vi "Analyze Pulse Waveform.vi"(0 "Waveform In":waveform(dbl)={"t0"=timestamp(3418839276.250478 s since 1904-01-01), "dt"=1e-06, "Y"=[5.0, 5.0, 9.0, 9.0, 9.0, 9.0, 9.0, 9.0, 9.0, 9.0, 5.0, 5.0, 5.0, 3.0, 3.0, 3.0, 3.0, 3.0, 3.0, 3.0, 3.0, 3.0, 3.0, 3.0, 3.0, 3.0, 3.0, 3.0, 3.0, 5.0, 5.0, 5.0, 5.0, 8.0, 8.0, 8.0, 8.0, 8.0, 8.0, 8.0, 8.0, 5.0, 5.0, 5.0, 3.0, 3.0, 3.0, 3.0, 3.0, 3.0, 3.0, 3.0, 3.0, 3.0, 3.0, 3.0, 3.0, 3.0, 3.0, 3.0, 5.0, 5.0, 5.0, 5.0, 0.0, 0.0, 0.0, 0.0, 0.0, 5.0, 5.0, 5.0, 5.0, 5.0, 5.0, 5.0, 5.0, 5.0, 5.0, 5.0, 5.0, 5.0, 5.0, 5.0, 5.0, 5.0, 5.0, 5.0, 5.0, 5.0, 5.0, 5.0, 5.0, 5.0, 5.0, 5.0, 5.0, 5.0, 5.0, 5.0, 5.0, 5.0, 9.0, 9.0, 9.0, 9.0, 9.0, 9.0, 9.0, 9.0, 5.0, 5.0, 5.0, 3.0, 3.0, 3.0, 3.0, 3.0, 3.0, 3.0, 3.0, 3.0, 3.0, 3.0, 3.0, 3.0, 3.0, 3.0, 3.0, 5.0, 5.0, 5.0, 5.0, 8.0, 8.0, 8.0, 8.0, 8.0, 8.0, 8.0, 8.0, 5.0, 5.0, 5.0, 3.0, 3.0, 3.0, 3.0, 3.0, 3.0, 3.0, 3.0, 3.0, 3.0, 3.0, 3.0, 3.0, 3.0, 3.0, 3.0, 5.0, 5.0, 5.0, 5.0, 0.0, 0.0, 0.0, 0.0, 0.0, 5.0, 5.0, 5.0, 5.0, 5.0, 5.0, 5.0, 5.0, 5.0, 5.0, 5.0, 5.0, 5.0, 5.0, 5.0, 5.0, 5.0, 5.0, 5.0, 5.0, 5.0, 5.0, 5.0, 5.0, 5.0, 5.0, 5.0, 5.0, 5.0, 5.0, 5.0, 5.0, 5.0, 9.0, 9.0, 9.0, 9.0, 9.0, 9.0, 9.0, 9.0, 5.0, 5.0, 5.0, 3.0, 3.0, 3.0, 3.0, 3.0, 3.0, 3.0, 3.0, 3.0, 3.0, 3.0, 3.0, 3.0, 3.0, 3.0, 3.0, 5.0, 5.0, 5.0, 5.0, 8.0, 8.0, 8.0, 8.0, 8.0, 8.0, 8.0, 8.0, 5.0, 5.0, 5.0, 3.0, 3.0, 3.0, 3.0, 3.0, 3.0, 3.0, 3.0, 3.0, 3.0, 3.0, 3.0, 3.0, 3.0, 3.0, 3.0, 5.0, 5.0, 5.0, 5.0, 0.0, 0.0, 0.0, 0.0, 0.0, 5.0, 5.0, 5.0, 5.0, 5.0, 5.0, 5.0, 5.0, 5.0, 5.0, 5.0, 5.0, 5.0, 5.0, 5.0, 5.0, 5.0, 5.0, 5.0, 5.0, 5.0, 5.0, 5.0, 5.0, 5.0, 5.0, 5.0, 5.0, 5.0, 5.0, 5.0, 5.0, 5.0, 9.0, 9.0, 9.0, 9.0, 9.0, 9.0, 9.0, 9.0, 5.0, 5.0, 5.0, 3.0, 3.0, 3.0, 3.0, 3.0, 3.0, 3.0, 3.0, 3.0, 3.0, 3.0, 3.0, 3.0, 3.0, 3.0, 3.0, 5.0, 5.0, 5.0, 5.0, 8.0, 8.0, 8.0, 8.0, 8.0, 8.0, 8.0, 8.0, 5.0, 5.0, 5.0, 3.0, 3.0, 3.0, 3.0, 3.0, 3.0, 3.0, 3.0, 3.0, 3.0, 3.0, 3.0, 3.0, 3.0, 3.0, 3.0, 5.0, 5.0, 5.0, 5.0, 0.0, 0.0, 0.0, 0.0, 0.0, 5.0, 5.0, 5.0, 5.0, 5.0, 5.0, 5.0, 5.0, 5.0, 5.0, 5.0, 5.0, 5.0, 5.0, 5.0, 5.0, 5.0, 5.0, 5.0, 5.0, 5.0, 5.0, 5.0, 5.0, 5.0, 5.0, 5.0, 5.0, 5.0, 5.0, 5.0, 5.0, 5.0, 9.0, 9.0, 9.0, 9.0, 9.0, 9.0, 9.0, 9.0, 5.0, 5.0, 5.0, 3.0, 3.0, 3.0, 3.0, 3.0, 3.0, 3.0, 3.0, 3.0, 3.0, 3.0, 3.0, 3.0, 3.0, 3.0, 3.0, 5.0, 5.0, 5.0, 5.0, 8.0, 8.0, 8.0, 8.0, 8.0, 8.0, 8.0, 8.0, 5.0, 5.0, 5.0, 3.0, 3.0, 3.0, 3.0, 3.0, 3.0, 3.0, 3.0, 3.0, 3.0, 3.0, 3.0, 3.0, 3.0, 3.0, 3.0, 5.0, 5.0, 5.0, 5.0, 0.0, 0.0, 0.0, 0.0, 0.0, 5.0, 5.0, 5.0, 5.0, 5.0, 5.0, 5.0, 5.0, 5.0, 5.0, 5.0, 5.0, 5.0, 5.0, 5.0, 5.0, 5.0, 5.0, 5.0, 5.0, 5.0, 5.0, 5.0, 5.0, 5.0, 5.0, 5.0, 5.0, 5.0, 5.0, 5.0, 5.0, 5.0, 5.0]}, 5 "Repetitions in the Input Waveform":i32, 7 "Pulse Characteristics":T1={"Pulses per Cycle"=2, "Load Resistance (Ohms)"=750.0, "Krec Value"=2, "Recovery Mode (T=Active)"=TRUE, "Target Stim Currents (Amps)"=[]}) -> (4 "Recovery Voltage":dbl[](array[numeric]), 6 "Recovery Holdoff Current":dbl[](array[numeric]), 8 "Interphase Delay Current":dbl[](array[numeric]), 10 "CBC Phase Voltage":dbl[](array[numeric]))   [LabVIEW 2010]
uses:
  <vilib>/measure/mamon.llb/Trigger Detection for 1 Channel.vi
  <vilib>/measure/NI_MAPro.lvlib
  <vilib>/Analysis/NI_AALBase.lvlib
panel:
  out "Normalized Waveform":waveform(dbl)(graph)
  # "The input waveform should be a capture of the STIM chip output\n(before the cap) when the output is held at 1/2 HVDD by the\nLoad Resistance.  This ensures that passive recovery and CBC\npulses are captured, because they look like pulses pulled to GND."
  # "The elements in these arrays correspond to the pulses per cycle.\nThey are the averages over all the repetitions in the waveform."
  # "Enter Target Current\nfor each in array below"
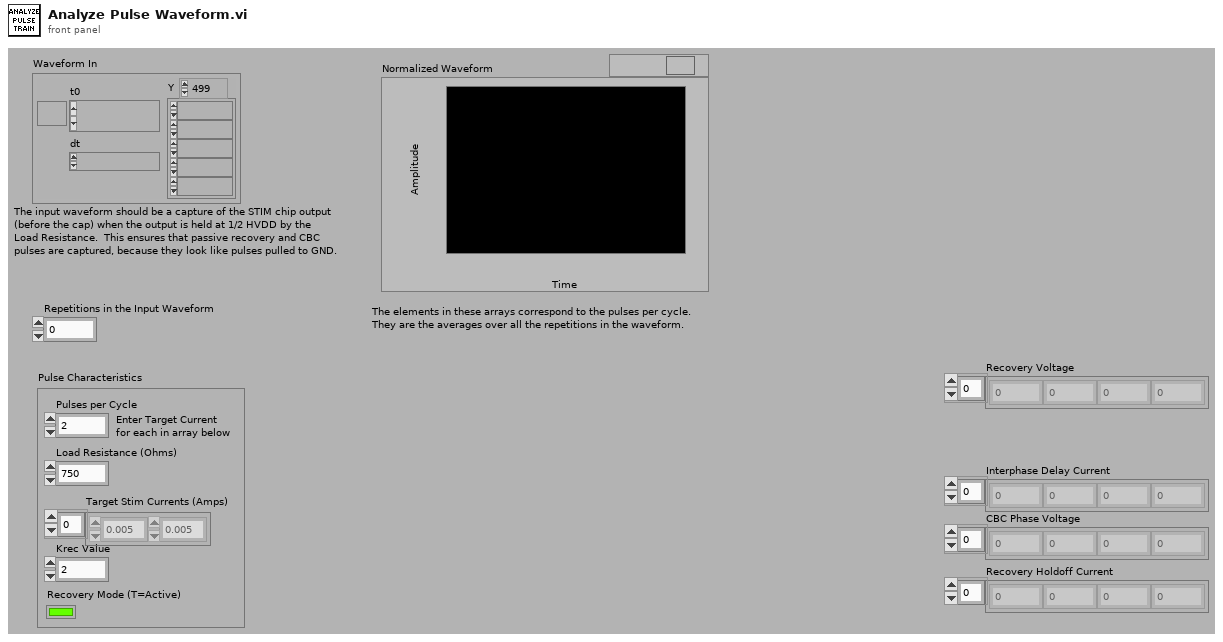
[diagram p1: front panel]
types:
  T1 = cluster{"Pulses per Cycle":i32, "Load Resistance (Ohms)":dbl, "Krec Value":i32, "Recovery Mode (T=Active)":bool, "Target Stim Currents (Amps)":dbl[]}
  T2 = cluster{"trigger slope":u16, "Trigger Level":dbl}[]
  T3 = cluster{"trigger slope":u16, "Trigger Level":dbl}
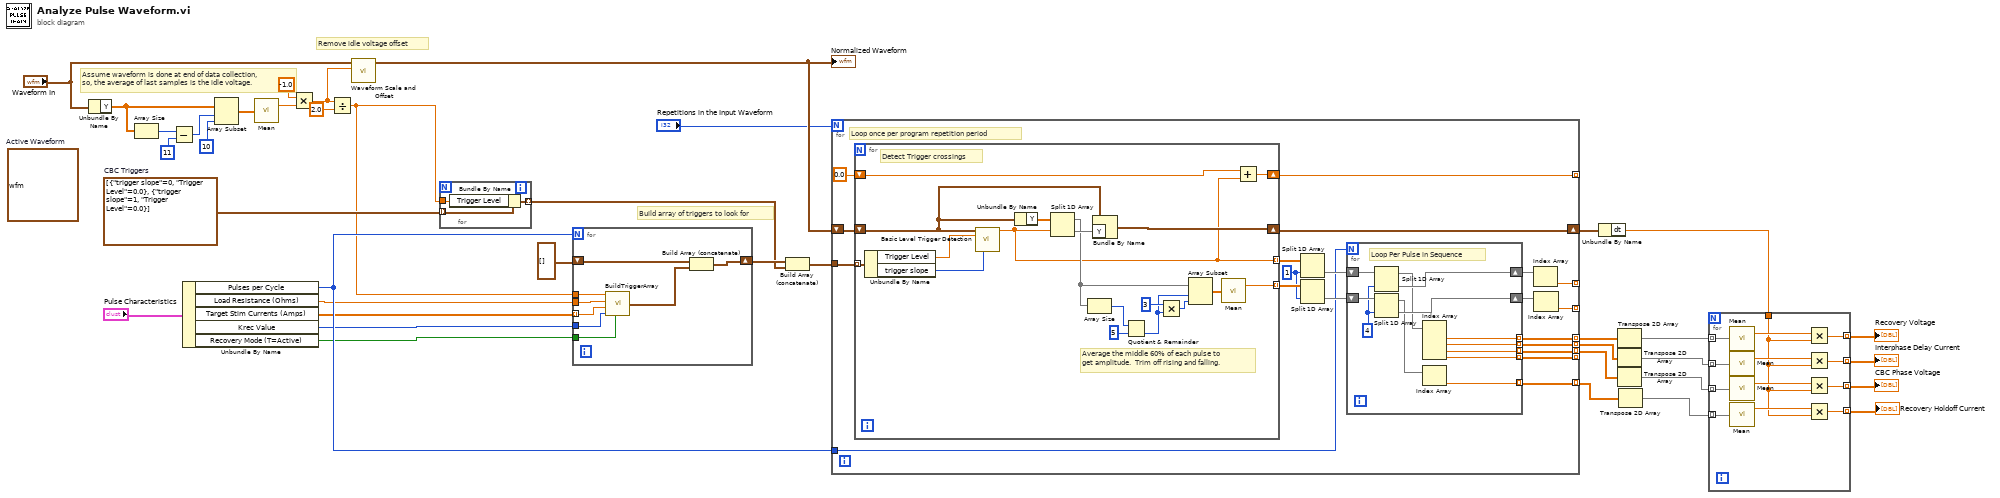
[diagram p0: block diagram]
diagram:
  (unwired) waveform(dbl) {"t0"=timestamp(3418839276.250478 s since 1904-01-01), "dt"=1e-06, "Y"=[5.0, 5.0, 9.0, 9.0, 9.0, 9.0, 9.0, 9.0, 9.0, 9.0, 5.0, 5.0, 5.0, 3.0, 3.0, 3.0, 3.0, 3.0, 3.0, 3.0, 3.0, 3.0, 3.0, 3.0, 3.0, 3.0, 3.0, 3.0, 3.0, 5.0, 5.0, 5.0, 5.0, 8.0, 8.0, 8.0, 8.0, 8.0, 8.0, 8.0, 8.0, 5.0, 5.0, 5.0, 3.0, 3.0, 3.0, 3.0, 3.0, 3.0, 3.0, 3.0, 3.0, 3.0, 3.0, 3.0, 3.0, 3.0, 3.0, 3.0, 5.0, 5.0, 5.0, 5.0, 0.0, 0.0, 0.0, 0.0, 0.0, 5.0, 5.0, 5.0, 5.0, 5.0, 5.0, 5.0, 5.0, 5.0, 5.0, 5.0, 5.0, 5.0, 5.0, 5.0, 5.0, 5.0, 5.0, 5.0, 5.0, 5.0, 5.0, 5.0, 5.0, 5.0, 5.0, 5.0, 5.0, 5.0, 5.0, 5.0, 5.0, 5.0, 9.0, 9.0, 9.0, 9.0, 9.0, 9.0, 9.0, 9.0, 5.0, 5.0, 5.0, 3.0, 3.0, 3.0, 3.0, 3.0, 3.0, 3.0, 3.0, 3.0, 3.0, 3.0, 3.0, 3.0, 3.0, 3.0, 3.0, 5.0, 5.0, 5.0, 5.0, 8.0, 8.0, 8.0, 8.0, 8.0, 8.0, 8.0, 8.0, 5.0, 5.0, 5.0, 3.0, 3.0, 3.0, 3.0, 3.0, 3.0, 3.0, 3.0, 3.0, 3.0, 3.0, 3.0, 3.0, 3.0, 3.0, 3.0, 5.0, 5.0, 5.0, 5.0, 0.0, 0.0, 0.0, 0.0, 0.0, 5.0, 5.0, 5.0, 5.0, 5.0, 5.0, 5.0, 5.0, 5.0, 5.0, 5.0, 5.0, 5.0, 5.0, 5.0, 5.0, 5.0, 5.0, 5.0, 5.0, 5.0, 5.0, 5.0, 5.0, 5.0, 5.0, 5.0, 5.0, 5.0, 5.0, 5.0, 5.0, 5.0, 9.0, 9.0, 9.0, 9.0, 9.0, 9.0, 9.0, 9.0, 5.0, 5.0, 5.0, 3.0, 3.0, 3.0, 3.0, 3.0, 3.0, 3.0, 3.0, 3.0, 3.0, 3.0, 3.0, 3.0, 3.0, 3.0, 3.0, 5.0, 5.0, 5.0, 5.0, 8.0, 8.0, 8.0, 8.0, 8.0, 8.0, 8.0, 8.0, 5.0, 5.0, 5.0, 3.0, 3.0, 3.0, 3.0, 3.0, 3.0, 3.0, 3.0, 3.0, 3.0, 3.0, 3.0, 3.0, 3.0, 3.0, 3.0, 5.0, 5.0, 5.0, 5.0, 0.0, 0.0, 0.0, 0.0, 0.0, 5.0, 5.0, 5.0, 5.0, 5.0, 5.0, 5.0, 5.0, 5.0, 5.0, 5.0, 5.0, 5.0, 5.0, 5.0, 5.0, 5.0, 5.0, 5.0, 5.0, 5.0, 5.0, 5.0, 5.0, 5.0, 5.0, 5.0, 5.0, 5.0, 5.0, 5.0, 5.0, 5.0, 9.0, 9.0, 9.0, 9.0, 9.0, 9.0, 9.0, 9.0, 5.0, 5.0, 5.0, 3.0, 3.0, 3.0, 3.0, 3.0, 3.0, 3.0, 3.0, 3.0, 3.0, 3.0, 3.0, 3.0, 3.0, 3.0, 3.0, 5.0, 5.0, 5.0, 5.0, 8.0, 8.0, 8.0, 8.0, 8.0, 8.0, 8.0, 8.0, 5.0, 5.0, 5.0, 3.0, 3.0, 3.0, 3.0, 3.0, 3.0, 3.0, 3.0, 3.0, 3.0, 3.0, 3.0, 3.0, 3.0, 3.0, 3.0, 5.0, 5.0, 5.0, 5.0, 0.0, 0.0, 0.0, 0.0, 0.0, 5.0, 5.0, 5.0, 5.0, 5.0, 5.0, 5.0, 5.0, 5.0, 5.0, 5.0, 5.0, 5.0, 5.0, 5.0, 5.0, 5.0, 5.0, 5.0, 5.0, 5.0, 5.0, 5.0, 5.0, 5.0, 5.0, 5.0, 5.0, 5.0, 5.0, 5.0, 5.0, 5.0, 9.0, 9.0, 9.0, 9.0, 9.0, 9.0, 9.0, 9.0, 5.0, 5.0, 5.0, 3.0, 3.0, 3.0, 3.0, 3.0, 3.0, 3.0, 3.0, 3.0, 3.0, 3.0, 3.0, 3.0, 3.0, 3.0, 3.0, 5.0, 5.0, 5.0, 5.0, 8.0, 8.0, 8.0, 8.0, 8.0, 8.0, 8.0, 8.0, 5.0, 5.0, 5.0, 3.0, 3.0, 3.0, 3.0, 3.0, 3.0, 3.0, 3.0, 3.0, 3.0, 3.0, 3.0, 3.0, 3.0, 3.0, 3.0, 5.0, 5.0, 5.0, 5.0, 0.0, 0.0, 0.0, 0.0, 0.0, 5.0, 5.0, 5.0, 5.0, 5.0, 5.0, 5.0, 5.0, 5.0, 5.0, 5.0, 5.0, 5.0, 5.0, 5.0, 5.0, 5.0, 5.0, 5.0, 5.0, 5.0, 5.0, 5.0, 5.0, 5.0, 5.0, 5.0, 5.0, 5.0, 5.0, 5.0, 5.0, 5.0, 5.0]}  # Active Waveform
  w27 = T2 [{"trigger slope"=0, "Trigger Level"=0.0}, {"trigger slope"=1, "Trigger Level"=0.0}]  # CBC Triggers
  # "Build array of triggers to look for"
  # "Remove idle voltage offset"
  # "Assume waveform is done at end of data collection,\nso, the average of last samples is the idle voltage."
  n1 = Unbundle By Name("Waveform In") -> ("Y"=w35:dbl[])
  n2 = Array Size(array=w35) -> (size(s)=w39:i32)
  n3 = Subtract(x=w39, y=11) -> (x-y=w37:i32)
  n4 = Unbundle By Name("Pulse Characteristics") -> ("Pulses per Cycle"=w15:i32, "Load Resistance (Ohms)"=w8:dbl, "Target Stim Currents (Amps)"=w12:dbl[], "Krec Value"=w11:i32, "Recovery Mode (T=Active)"=w13:bool)
  n5 = Array Subset(array=w35, index=w37, length=10 ("index")) -> (w34:dbl[])
  n6 = call <vilib>:"Mean.vi"("X"=w34) -> ("mean"=w33:dbl)  [unwired: 1 out]
  n7 = Multiply(x=-1.0, y=w33) -> (x*y=w26:dbl)
  n8 = Divide(x=w26, y=2.0) -> (x/y=w14:dbl)
  n9 = call <vilib>:"Waveform Scale and Offset.vi"("offset"=w26, "waveform in"="Waveform In") -> ("waveform out"=w22:waveform(dbl))  [unwired: 8 in, 1 out]
  "Normalized Waveform" <- w22
  n10 = for {
    tunnel: w27 -> [w42] mode=indexing
    tunnel: w14 -> [w41]
    tunnel: [w40] -> w24 mode=indexing
    n11 = Bundle By Name(cluster=w42, "Trigger Level"=w41) -> (w40:T3)
  }
  n12 = for {
    N: w15 -> [_]
    shift-right: [w50] -> w28
    shift-left: T2 [] -> [w49]
    tunnel: w14 -> [w48]
    tunnel: w13 -> [w47]
    tunnel: w8 -> [w46]
    tunnel: w12 -> [w45] mode=indexing
    tunnel: w11 -> [w44]
    n13 = call "BuildTriggerArray.vi"("CBC Trigger Level"=w48, "Load Resistance (Ohms)"=w46, "Target Stim Current (Amps)"=w45, "Krec Value"=w44, "Recovery Mode (T=Active)"=w47) -> ("Pulse Triggers"=w43:T2)
    n14 = Build Array (concatenate)(w49, w43) -> (w50:T2)
  }
  n15 = Build Array (concatenate)(w28, w24) -> (w23:T2)
  n16 = for {
    N: "Repetitions in the Input Waveform" -> [_]
    tunnel: w23 -> [w70]
    shift-right: [w66] -> w9
    shift-left: w22 -> [w69]
    tunnel: w15 -> [w63]
    tunnel: [w60] -> _ mode=indexing
    tunnel: [w59] -> _ mode=indexing
    tunnel: [w58] -> w21 mode=indexing
    tunnel: [w57] -> w20 mode=indexing
    tunnel: [w56] -> w19 mode=indexing
    tunnel: [w55] -> _ mode=indexing
    tunnel: [w52] -> _ mode=indexing
    tunnel: [w51] -> w1 mode=indexing
    w67 = 1 ("index")
    # "Loop once per program repetition period"
    n17 = for {
      tunnel: w70 -> [w100] mode=indexing
      shift-right: [w86] -> w66
      shift-left: w69 -> [w95]
      tunnel: [w87] -> w68 mode=indexing
      tunnel: [w83] -> w53 mode=indexing
      shift-right: [w85] -> w52
      shift-left: 0.0 -> [w84]
      # "Detect Trigger crossings"
      # "Average the middle 60% of each pulse to\nget amplitude.  Trim off rising and falling."
      n18 = Unbundle By Name(w100) -> ("Trigger Level"=w99:dbl, "trigger slope"=w98:u16)
      n19 = call-poly <vilib>:"Basic Level Trigger Detection.vi"("signal in"=w95, "level"=w99, "trigger slope"=w98) -> ("trigger location"=w83:dbl)  [unwired: 10 in, 2 out]
      n20 = Unbundle By Name(w95) -> ("Y"=w97:dbl[])
      n21 = Split 1D Array(array=w97, index=w83) -> (first subarray=w89:dbl[], second subarray=w96:dbl[])
      n22 = Array Size(array=w89) -> (size(s)=w94:i32)
      n23 = Bundle By Name(cluster=w95, "Y"=w96) -> (w86:waveform(dbl))
      n24 = Quotient & Remainder(x=w94, y=5) -> (floor(x/y)=w91:i32)  [unwired: 1 out]
      n25 = Multiply(x=3, y=w91) -> (x*y=w90:i32)
      n26 = Array Subset(array=w89, index=w91, length=w90) -> (w88:dbl[])
      n27 = call <vilib>:"Mean.vi"("X"=w88) -> ("mean"=w87:dbl)  [unwired: 1 out]
      n28 = Add(x=w84, y=w83) -> (x+y=w85:dbl)
    }
    n29 = Split 1D Array(array=w53, index=w67) -> (second subarray=w65:dbl[])  [unwired: 1 out]
    n30 = Split 1D Array(array=w68, index=w67) -> (second subarray=w64:dbl[])  [unwired: 1 out]
    n31 = for {
      N: w63 -> [_]
      shift-right: [w80] -> w62
      shift-left: w65 -> [w82]
      shift-right: [w79] -> w61
      shift-left: w64 -> [w81]
      tunnel: [w77] -> w58 mode=indexing
      tunnel: [w76] -> w57 mode=indexing
      tunnel: [w75] -> w56 mode=indexing
      tunnel: [w74] -> w55 mode=indexing
      tunnel: [w71] -> w51 mode=indexing
      w73 = 4 ("index")
      # "Loop Per Pulse in Sequence"
      n32 = Split 1D Array(array=w82, index=w73) -> (first subarray=w78:dbl[], second subarray=w80:dbl[])
      n33 = Split 1D Array(array=w81, index=w73) -> (first subarray=w72:dbl[], second subarray=w79:dbl[])
      n34 = Index Array(array=w78) -> (element #1=w77:dbl, element #2=w76:dbl, element #3=w75:dbl, element #4=w74:dbl)  [unwired: 4 in]
      n35 = Index Array(array=w72) -> (element=w71:dbl)  [unwired: 1 in]
    }
    n36 = Index Array(array=w62) -> (element=w60:dbl)  [unwired: 1 in]
    n37 = Index Array(array=w61) -> (element=w59:dbl)  [unwired: 1 in]
  }
  n38 = Unbundle By Name(w9) -> ("dt"=w7:dbl)
  n39 = Transpose 2D Array(2D array=w21) -> (transposed array=w18:dbl[][])
  n40 = Transpose 2D Array(2D array=w20) -> (transposed array=w17:dbl[][])
  n41 = Transpose 2D Array(2D array=w19) -> (transposed array=w16:dbl[][])
  n42 = Transpose 2D Array(2D array=w1) -> (transposed array=w3:dbl[][])
  n43 = for {
    tunnel: w18 -> [w113] mode=indexing
    tunnel: w17 -> [w112] mode=indexing
    tunnel: w16 -> [w111] mode=indexing
    tunnel: [w110] -> w6 mode=indexing
    tunnel: [w109] -> w4 mode=indexing
    tunnel: [w108] -> w5 mode=indexing
    tunnel: w7 -> [w103]
    tunnel: w3 -> [w102] mode=indexing
    tunnel: [w101] -> w2 mode=indexing
    n44 = call <vilib>:"Mean.vi"("X"=w113) -> ("mean"=w107:dbl)  [unwired: 1 out]
    n45 = call <vilib>:"Mean.vi"("X"=w112) -> ("mean"=w106:dbl)  [unwired: 1 out]
    n46 = call <vilib>:"Mean.vi"("X"=w111) -> ("mean"=w105:dbl)  [unwired: 1 out]
    n47 = call <vilib>:"Mean.vi"("X"=w102) -> ("mean"=w104:dbl)  [unwired: 1 out]
    n48 = Multiply(x=w107, y=w103) -> (x*y=w110:dbl)
    n49 = Multiply(x=w106, y=w103) -> (x*y=w109:dbl)
    n50 = Multiply(x=w105, y=w103) -> (x*y=w108:dbl)
    n51 = Multiply(x=w104, y=w103) -> (x*y=w101:dbl)
  }
  "Recovery Voltage" <- w6
  "Interphase Delay Current" <- w4
  "CBC Phase Voltage" <- w5
  "Recovery Holdoff Current" <- w2
